vi "Get SMO Public API.vi"(8 "error in (no error)":errorcluster, 11 "RP100 in":refnum<class "RP100.lvclass">) -> (0 "error out":errorcluster, 2 "Commands":string[](array[string]), 3 "RP100 out":refnum<class "RP100.lvclass">)   [LabVIEW 2019, in "RP100.lvclass"]
uses:
  RP100.lvclass
  Typedefs/Commands--Enum.ctl
  <userlib>/LevyLab/Instrument Framework/Instrument Types/Strain/Instrument.Strain.lvclass
  <userlib>/LevyLab/Instrument Framework/SMOs/Instrument/Instrument.lvclass
panel:
  in  "Commands":T1
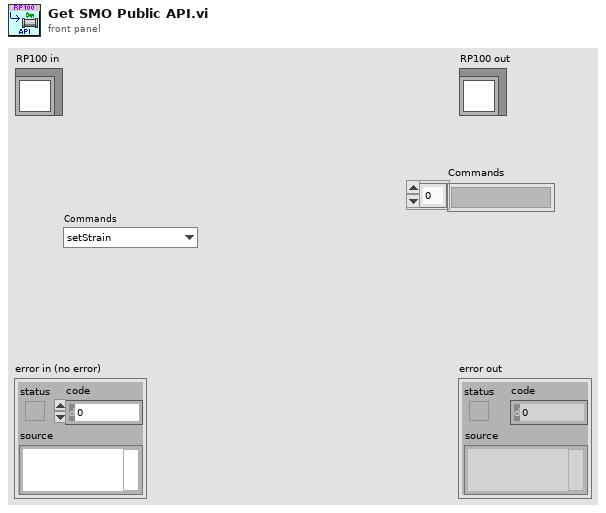
[diagram p1: front panel]
types:
  T1 = typedef "RP100.lvclass/Commands--Enum.ctl" = enum16{"setStrain", "getStrain", "setLevel", "getLevel"}
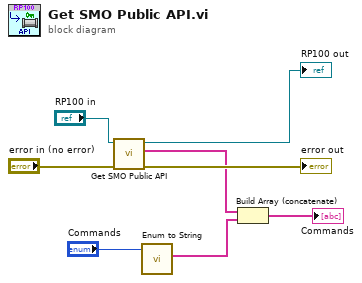
[diagram p0: block diagram]
diagram:
  n1 = call-parent "Get SMO Public API.vi"("error in (no error)"="error in (no error)", "Instrument in"="RP100 in") -> ("error out"=→"error out":errorcluster, "Commands"=w3:string[], "Instrument out"=→"RP100 out":refnum<class "RP100.lvclass">)  [unwired: 7 in]
  n2 = call <userlib>:"Enum to String.vi"("Command"="Commands") -> ("Commands []"=w4:string[])  [unwired: 9 in, 1 out]
  n3 = Build Array (concatenate)(w3, w4) -> (→"Commands":string[])
